vi "get Origin and Angle.vi"(11 "Origin and Axis path":path) -> (2 "angle radian":dbl, 3 "Origin":dbl[](array[numeric]))   [LabVIEW 2016]
uses:
  <vilib>/Utility/file.llb/Read Delimited Spreadsheet (DBL).vi
panel:
  out "angle degress":dbl
  out "all rows":dbl[][](array[numeric])
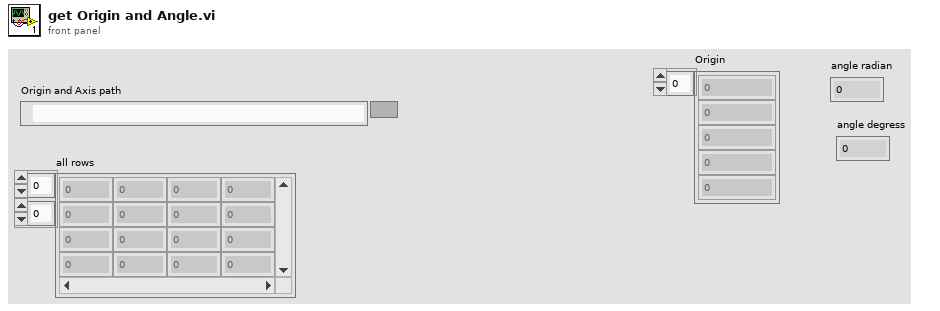
[diagram p1: front panel]
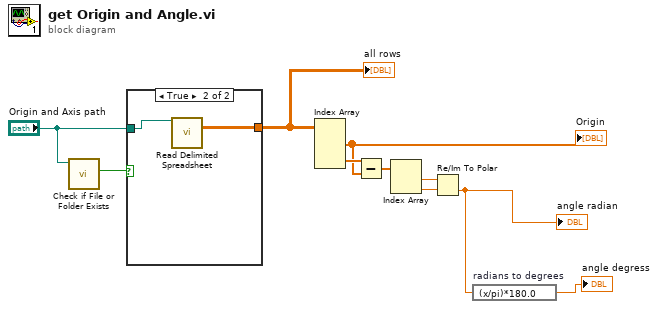
[diagram p0: block diagram]
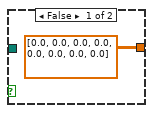
[diagram p2: hidden frame]
diagram:
  n1 = call <vilib>:"Check if File or Folder Exists.vi"("path"="Origin and Axis path") -> ("file or folder exists?"=w1:bool)  [unwired: 8 in, 2 out]
  n2 = case shown="True" w1 {
    tunnel: [dbl[][] [[0.0, 0.0, 0.0, 0.0], [0.0, 0.0, 0.0, 0.0]] ("all rows") w13] -> w5
    tunnel: "Origin and Axis path" -> [_ w12]
    frame False {
    }
    frame True {
      n3 = call-poly <vilib>:"Read Delimited Spreadsheet.vi"("file path (dialog if empty)"=w12) -> ("all rows"=w13:dbl[][])  [unwired: 9 in, 5 out]
    }
  }
  "all rows" <- w5
  n4 = Index Array(array=w5) -> (element #1=w7:dbl[], element #2=w8:dbl[])  [unwired: 4 in]
  "Origin" <- w7
  n5 = Subtract(x=w8, y=w7) -> (x-y=w6:dbl[])
  n6 = Index Array(array=w6) -> (element #1=w10:dbl, element #2=w9:dbl)  [unwired: 2 in]
  n7 = Re/Im To Polar(2:w9, 3:w10) -> (0:w4:dbl)  [unwired: 1 out]
  "angle radian" <- w4
  n8 = expression code="(x/pi)*180.0" "radians to degrees"(w4) -> (→"angle degress":dbl)
